vi "Main.vi"() -> ()   [LabVIEW 2018]
uses:
  <vilib>/DAQmx/read.llb/DAQmx Read (Analog 2D DBL NChan NSamp).vi
panel:
  out "Powers":dbl[](array[numeric])=[100.0, 150.0, 200.0, 250.0]
  out "Voltages":dbl[](array[numeric])=[2.5, 2.75, 3.0]
  in  "Min_Voltage [V]":dbl=2.5 format="%0.2f"
  in  "Max_Voltage [V]":dbl=3.0 format="%0.2f"
  in  "N_Voltage":i32=3
  out "fc - Sampling frequency \nof the card":dbl=50000.0
  in  "Number of Analysis":i32=31
  out "Load \nGenerating":i32=250
  out "Voltage \nGenerating":dbl=3.0
  in  "N_Power":i32=4
  out "fs - Detected frequency \nof the signal":dbl=231.43662913014396
  in  "Np_Analysis":i32=5
  in  "stop":bool
  in  "VISA Chroma (Load)":refnum<visa-resource-name>="GPIB0::1::INSTR"
  in  "Max_Power [W]":dbl=250.0 format="%0.2f"
  in  "Min_Power [W]":dbl=100.0 format="%0.2f"
  in  "Generation Channels":tag="cDAQ9188XT-1947DFEMod5/ao0"
  in  "Current Acquisition Channels":tag="cDAQ9188XT-1947DFEMod1/ai0:2"
  in  "Voltage Acquisition Channels":tag="cDAQ9188XT-1947DFEMod2/ai0:2, cDAQ9188XT-1947DFEMod8/ai2:1, cDAQ9188XT-1947DFEMod4/ai3:2"
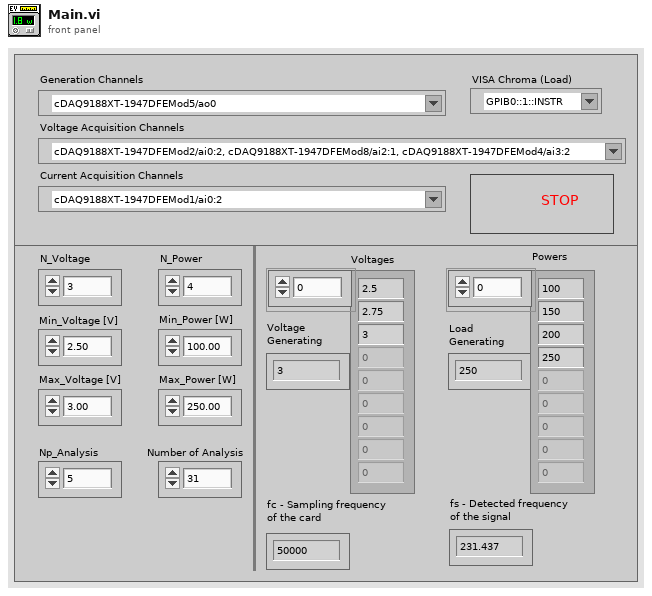
[diagram p1: front panel]
types:
  T1 = typedef "array misure.ctl" = cluster{"fase R ":T2, "fase  S":T2, "fase T":T2, "Input":T2, "output":T2, "Fc (Frequenza di campionamneto":dbl}
  T2 = typedef "coppie.ctl" = cluster{"V":dbl[], "I":dbl[]}
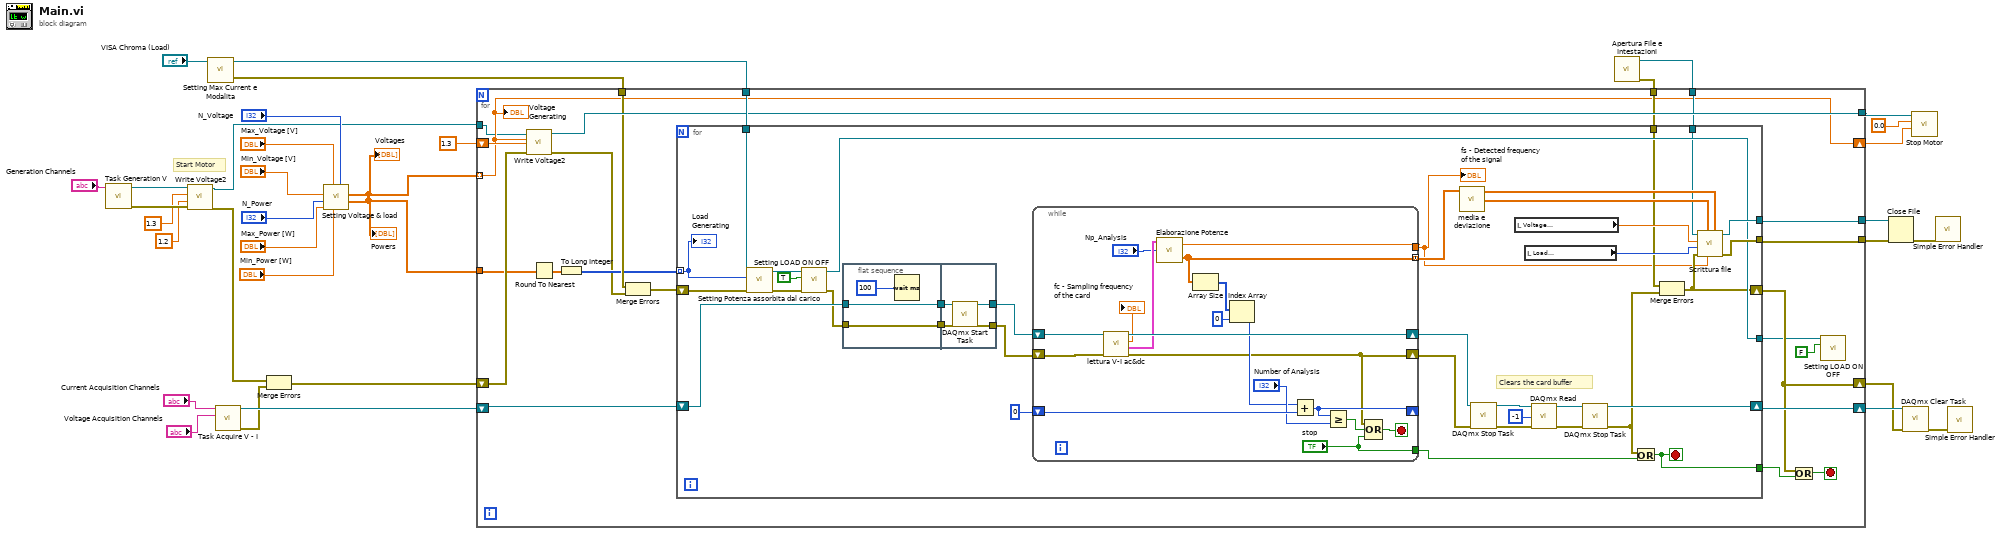
[diagram p0: block diagram]
diagram:
  # "Start Motor"
  n1 = call "Task Generation V.vi"("Generation Channels"="Generation Channels") -> ("error out"=w9:errorcluster, "Refnum out"=w8:refnum<k21>)  [unwired: 9 in]
  n2 = call "Write Voltage2.vi"("error in (no error)"=w9, "Current voltage"=1.2 ("current voltage"), "Desired voltage"=1.3 ("desired voltage"), "Refnum in"=w8) -> ("error out"=w6:errorcluster, "Refnum out"=w7:refnum<k21>)  [unwired: 6 in]
  n3 = call "Setting Max Current e Modalita.vi"("VISA resource name"="VISA Chroma (Load)") -> ("VISA resource name out"=w27:refnum<visa-resource-name>, "error out"=w26:errorcluster)  [unwired: 6 in]
  n4 = call "Task Acquire V - I.vi"("Voltage Acquisition Channels"="Voltage Acquisition Channels", "Current Acquisition Channels"="Current Acquisition Channels") -> ("error out"=w29:errorcluster, "Refnum out"=w35:refnum<k21>)  [unwired: 8 in]
  n5 = Merge Errors(w6, w29) -> (w28:errorcluster)
  n6 = call "Setting Voltage & load.vi"("N_Voltage"="N_Voltage", "Min_Power [W]"="Min_Power [W]", "Max_Voltage [V]"="Max_Voltage [V]", "Max_Power [W]"="Max_Power [W]", "N_Power"="N_Power", "Min_Voltage [V]"="Min_Voltage [V]") -> ("Powers"=w11:dbl[], "Voltages"=w12:dbl[])  [unwired: 4 in]
  "Voltages" <- w12
  "Powers" <- w11
  n7 = call "Apertura File e Intestazioni.vi"() -> ("error out 2"=w15:errorcluster, "Byte Stream File out"=w16:refnum<file>)  [unwired: 10 in]
  n8 = for {
    shift-right: [w57] -> w33
    shift-left: w35 -> [w58]
    shift-right: [w49] -> w21
    shift-left: w28 -> [w55]
    tunnel: w11 -> [w47]
    tunnel: w27 -> [w56]
    tunnel: w26 -> [w46]
    tunnel: w12 -> [w37] mode=indexing
    tunnel: w7 -> [w36]
    tunnel: [w54] -> w3
    tunnel: [w53] -> w24
    tunnel: [w52] -> w23
    tunnel: w16 -> [w41]
    tunnel: w15 -> [w40]
    shift-right: [w37] -> w1
    shift-left: 1.3 -> [w38]
    stop <- w51 stop-if-true
    n9 = call "Write Voltage2.vi"("error in (no error)"=w55, "Current voltage"=w38, "Desired voltage"=w37, "Refnum in"=w36) -> ("error out"=w39:errorcluster, "Refnum out"=w54:refnum<k21>)  [unwired: 6 in]
    n10 = Round To Nearest(number=w47) -> (nearest integer value=w48:dbl[])
    n11 = To Long Integer(number=w48) -> (32bit integer=w45:i32[])
    n12 = Merge Errors(w46, w39) -> (w44:errorcluster)
    n13 = for {
      shift-right: [w69] -> w57
      shift-left: w58 -> [w94]
      shift-right: [w64] -> w49
      shift-left: w44 -> [w76]
      tunnel: w56 -> [w89]
      tunnel: [w80] -> w50
      tunnel: [w83] -> w53
      tunnel: [w82] -> w52
      tunnel: w45 -> [w77] mode=indexing
      tunnel: [w65] -> w42
      tunnel: w41 -> [w63]
      tunnel: w40 -> [w61]
      stop <- w80 stop-if-true
      # "Clears the card buffer"
      n14 = call "Setting Potenza assorbita dal carico.vi"("error in (no error)"=w76, "POWER [WATT]"=w77, "VISA resource name"=w89) -> ("error out"=w90:errorcluster, "VISA resource name out"=w87:refnum<visa-resource-name>)  [unwired: 6 in]
      n15 = call "Setting LOAD ON OFF.vi"("error in (no error)"=w90, "ON/OFF"=TRUE ("Boolean"), "VISA resource name"=w87) -> ("error out"=w88:errorcluster, "VISA resource name out"=w65:refnum<visa-resource-name>)  [unwired: 5 in]
      n16 = flat-sequence {
        tunnel: w88 -> [w96]
        tunnel: w94 -> [w97]
        tunnel: [w97] -> w79
        tunnel: [w96] -> w78
        tunnel: [w100] -> w93
        tunnel: [w99] -> w92
        tunnel: w79 -> [w101]
        tunnel: w78 -> [w98]
        frame #0 {
          n17 = Wait (ms)(milliseconds to wait=u32 100) -> ()  [unwired: 1 out]
        }
        frame #1 {
          n18 = call <vilib>:"DAQmx Start Task.vi"("task/channels in"=w101, "error in"=w98) -> ("task out"=w100:refnum<k21>, "error out"=w99:errorcluster)  [unwired: 12 in]
        }
      }
      n19 = while {
        shift-right: [w114] -> w91
        shift-left: w93 -> [w119]
        shift-right: [w105] -> w75
        shift-left: w92 -> [w118]
        tunnel: ["stop"] -> w86
        tunnel: [w111] -> w60
        shift-right: [w115] -> _
        shift-left: 0 -> [w117]
        tunnel: [w110] -> w68 mode=concatenating
        stop <- w102 stop-if-true
        n20 = call "lettura V-I ac&dc.vi"("error in (no error)"=w118, "Refnum in"=w119) -> ("error out"=w105:errorcluster, "Cluster"=w113:T1, "fc - Sampling frequency \nof the card"=→"fc - Sampling frequency \nof the card":dbl, "Refnum out"=w114:refnum<k21>)  [unwired: 6 in]
        n21 = call "Elaborazione Potenze.vi"("Np_Analysis"="Np_Analysis", "Cluster"=w113) -> ("transposed array"=w110:dbl[][], "fs - Detected frequency \nof the signal"=w111:dbl)  [unwired: 2 in]
        n22 = Array Size(array=w110) -> (size(s)=w109:i32[])
        n23 = Index Array(array=w109, index=0) -> (element=w107:i32)
        n24 = Add(x=w107, y=w117) -> (x+y=w115:i32)
        n25 = Greater Or Equal?(x=w115, y="Number of Analysis") -> (x >= y?=w104:bool)
        n26 = Compound Arithmetic op=OR(w105, w104, "stop") -> (w102:bool)
      }
      "fs - Detected frequency \nof the signal" <- w60
      n27 = call "media e deviazione.vi"("2D array"=w68) -> ("Mean Array - Active Power"=w67:dbl[], "Dev Array - Active Power"=w66:dbl[])  [unwired: 6 in]
      n28 = call <vilib>:"DAQmx Stop Task.vi"("task/channels in"=w91, "error in"=w75) -> ("task out"=w73:refnum<k21>, "error out"=w74:errorcluster)  [unwired: 12 in]
      n29 = local read "Voltage \nGenerating"() -> (w85:dbl)
      n30 = local read "Load \nGenerating"() -> (w84:i32)
      n31 = call-poly <vilib>:"DAQmx Read.vi"("task/channels in"=w73, "number of samples per channel"=-1, "error in"=w74) -> ("task out"=w71:refnum<k21>, "error out"=w70:errorcluster)  [unwired: 10 in, 1 out]
      n32 = call <vilib>:"DAQmx Stop Task.vi"("task/channels in"=w71, "error in"=w70) -> ("task out"=w69:refnum<k21>, "error out"=w62:errorcluster)  [unwired: 12 in]
      n33 = Or(x=w62, y=w86) -> (x .or. y?=w80:bool)
      n34 = Merge Errors(w61, w62) -> (w64:errorcluster)
      n35 = call "Scrittura file.vi"("Mean Array"=w67, "Frequency"=w60, "Dev. Array"=w66, "error in (no error)"=w64, "Load"=w84, "Voltage"=w85, "Byte Stream File in"=w63) -> ("error out"=w82:errorcluster, "Byte Stream File out"=w83:refnum<file>)  [unwired: 3 in]
      "Load \nGenerating" <- w77
    }
    n36 = Or(x=w49, y=w50) -> (x .or. y?=w51:bool)
    n37 = call "Setting LOAD ON OFF.vi"("ON/OFF"=FALSE ("Boolean"), "VISA resource name"=w42) -> ()  [unwired: 6 in, 2 out]
    "Voltage \nGenerating" <- w37
  }
  n38 = Close File(refnum=w24, error in=w23) -> (error out=w22:errorcluster)  [unwired: 1 out]
  n39 = call <vilib>:"DAQmx Clear Task.vi"("task in"=w33, "error in"=w21) -> ("error out"=w34:errorcluster)  [unwired: 13 in]
  n40 = call "Stop Motor.vi"("Current voltage"=w1, "Desired voltage"=0.0 ("desired voltage"), "Refnum in"=w3) -> ()  [unwired: 9 in]
  n41 = call <vilib>:"Simple Error Handler.vi"("error in (no error)"=w22) -> ()  [unwired: 4 in, 5 out]
  n42 = call <vilib>:"Simple Error Handler.vi"("error in (no error)"=w34) -> ()  [unwired: 4 in, 5 out]
